vi "MT Format Eye Diagram.vi"   [LabVIEW 2020, in "niDMT.lvlib"]
doc: "Specifies a complex- or real-valued waveform, divides it into segments, and displays those segments as plots on a waveform graph. This VI determines the segment length based on the <B>symbol rate</B> and <B>eye length</B> parameters."
uses:
  <vilib>/addons/Modulation/niDMT.lvlib
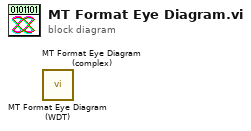
[diagram p0: block diagram]
diagram:
  n1 = call <vilib>:"MT Format Eye Diagram (WDT).vi"() -> ()  [unwired: 14 in, 2 out]
  n2 = call <vilib>:"MT Format Eye Diagram (complex).vi"() -> ()  [unwired: 14 in, 2 out]
